vi "Close API Reference.vi"(8 "error in (no error)":errorcluster, 11 "Execution API In":refnum<class "Execution API.lvclass">) -> (0 "error out":errorcluster)   [LabVIEW 2020, in "Execution API.lvclass"]
doc: "Closes the API reference. Please note that any Event Registrations obtained from the Register for Events.vi will need to be unregistered for."
uses:
  Execution API.lvclass
  Execution API.lvclass/Execution API.ctl
  Framework/Plugin/Plugin.lvclass
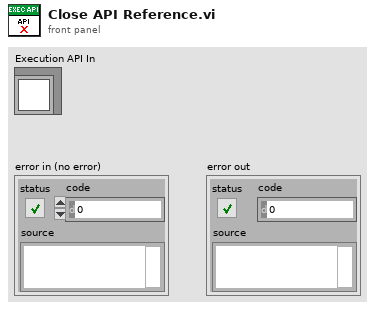
[diagram p1: front panel]
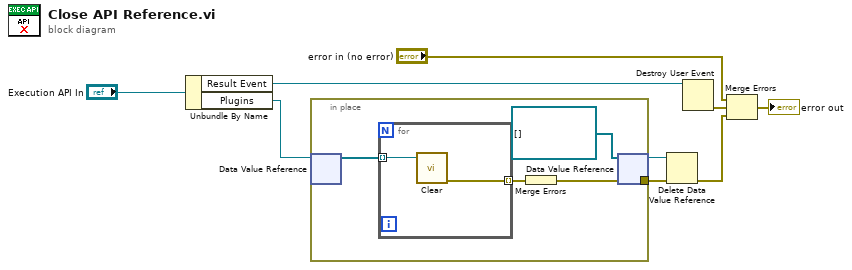
[diagram p0: block diagram]
diagram:
  n1 = Unbundle By Name("Execution API In") -> ("Result Event"=w6:refnum<user-event>, "Plugins"=w3:refnum<data-value>)
  n2 = in-place {
    in-place-border: [w11] -> w4
    n3 = in-place-dvr #1(w3) -> (w12:refnum<class "Plugin.lvclass">[])  [unwired: 1 out]
    n4 = for {
      tunnel: w12 -> [w15] mode=indexing
      tunnel: [w14] -> w13 mode=indexing
      n5 = call-dynamic "Clear.vi"("Plugin in"=w15) -> ("error out"=w14:errorcluster)  [unwired: 10 in]
    }
    n6 = Merge Errors(w13) -> (w11:errorcluster)
    n7 = in-place-dvr #1(refnum<class "Plugin.lvclass">[] [] ("data value")) -> (w1:refnum<data-value>)  [unwired: 1 out]
  }
  n8 = Delete Data Value Reference(data value reference=w1, error in=w4) -> (error out=w2:errorcluster)  [unwired: 1 out]
  n9 = Destroy User Event(user event=w6) -> (error out=w5:errorcluster)  [unwired: 1 in]
  n10 = Merge Errors("error in (no error)", w5, w2) -> (→"error out":errorcluster)
